vi "Remove form.vi"(8 "error in (no error)":errorcluster, 10 "Form ID":T1, 11 "Update Fields Logic in":refnum<class "Update Fields Logic.lvclass">) -> (0 "error out":errorcluster, 3 "Update Fields Logic out":refnum<class "Update Fields Logic.lvclass">)   [LabVIEW 2020, in "Form Server Interfaces.lvlib" / "Update Fields Logic.lvclass"]
uses:
  Update Fields Logic.lvclass
  Form ID.ctl
  Form Server Interfaces.lvlib
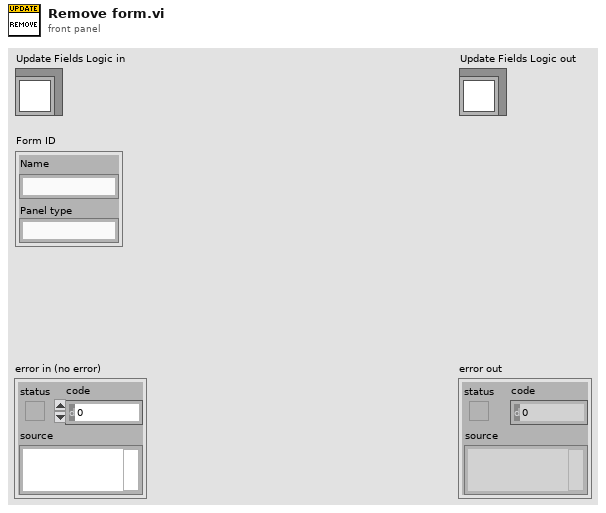
[diagram p1: front panel]
types:
  T1 = typedef "Form Server Interfaces.lvlib/Form ID.ctl" = cluster{"Name":string, "Panel type":string}
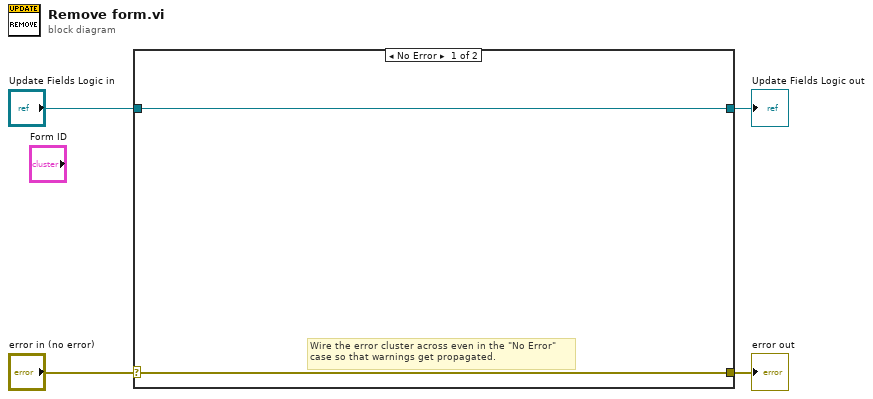
[diagram p0: block diagram]
diagram:
  n1 = case shown="No Error" "error in (no error)" {
    selector: "error in (no error)" -> [w5 w8]
    tunnel: [w5 w8] -> w3
    tunnel: [w6 w7] -> w1
    tunnel: "Update Fields Logic in" -> [w6 w7]
    frame No Error {
      # "Wire the error cluster across even in the \"No Error\"\ncase so that warnings get propagated."
    }
    frame Error {
    }
  }
  "error out" <- w3
  "Update Fields Logic out" <- w1
